vi "DIO Write Init.vi"(1 "device":i16=1) -> (0 "task ID out":u32)   [LabVIEW 2009]
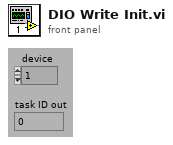
[diagram p1: front panel]
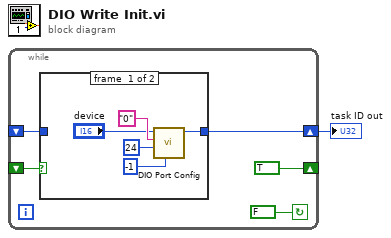
[diagram p0: block diagram]
diagram:
  n1 = while {
    shift-left: _ -> [w2]
    shift-right: [w3] -> w1
    shift-left: _ -> [w5]
    shift-right: [TRUE] -> _
    stop <- FALSE continue-if-true
    n2 = case shown="False" w5 {
      tunnel: [w7 w12] -> w3
      tunnel: w2 -> [_ w12]
      frame #0 {
        n3 = call <vilib>:"DIO Port Config.vi"("line direction map"=-1, "port width"=i16 24, "digital channel"="0", "device"="device") -> ("task ID out"=w7:u32)  [unwired: 6 in, 1 out]
      }
      frame #1 {
      }
    }
  }
  "task ID out" <- w1
